vi "configuration UI.vi"() -> ()   [LabVIEW 2013, in "user tag bus module editor node.lvclass"]
uses:
  user tag bus module editor node.lvclass
  <vilib>/CEF_TreeControl/Node/NodeRef.ctl
  <vilib>/CEF_TreeControl/Node/NISE_CEF_Node.lvclass
  <vilib>/NI/AMC/Message Queue.ctl
  <vilib>/NI/AMC/Message.ctl
  <vilib>/NI/Tools/Keyed Array/KeyedArray.ctl
  <vilib>/CEF_TreeControl/Node/UserEventRef.ctl
  <vilib>/CEF_TreeControl/Controls/EventCluster.ctl
  module/configuration/state module configuration.ctl
  <vilib>/NI/Tag Bus Module Framework/channel/TBM channel.lvclass
  user tag bus module editor node.lvclass/user tag bus module editor node.ctl
  <vilib>/NI/Tag Bus Module Framework/root configuration/TBM configuration.lvclass/TBM configuration.ctl
  module/configuration/user tag bus module configuration.lvclass/user tag bus module configuration.ctl
  <vilib>/NI/Tag Bus Module Framework/root configuration/create GUID.vi
  module/configuration/user tag bus module configuration.lvclass
  <vilib>/CEF_TreeControl/NISE_CEF_TreeControl.lvlib
  Configuration Editor/Classes/Engine Parent/Engine Parent Editor Node.lvclass
  <vilib>/NI/Tag Bus Module Framework/root configuration/TBM configuration.lvclass
  <vilib>/NI/Tools/Keyed Array/Tools_KeyedArray.lvlib
  <vilib>/NI/AMC/AMC.lvlib
panel:
  in  "Tab Control":enum32{"Static State Configuration"}(tab)
  in  "Output Tag":u16(ring)
  in  "Input Tag":u16(ring)
  in  "Initial State":u8
  in  "user event":T1
  in  "main queue":T2
  in  "node ref":T3
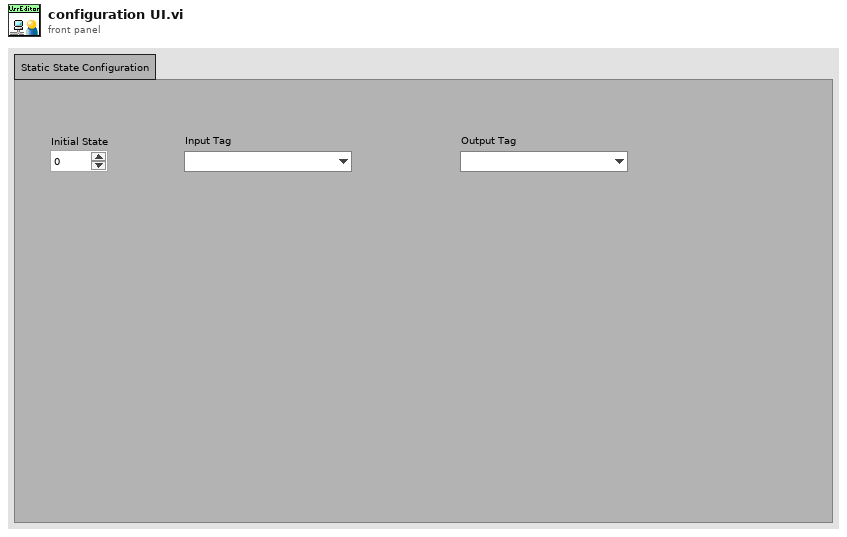
[diagram p1: front panel]
types:
  T1 = typedef "NISE_CEF_Node.lvclass/UserEventRef.ctl" = refnum<user-event>
  T2 = typedef "AMC.lvlib/Message Queue.ctl" = refnum<queue>
  T3 = typedef "NISE_CEF_Node.lvclass/NodeRef.ctl" = refnum<data-value>
  T4 = typedef "NISE_CEF_TreeControl.lvlib/EventCluster.ctl" = cluster{"command":string, "data":string}
  T5 = typedef "user tag bus module configuration.lvclass/state module configuration.ctl" = cluster{"fixed input":refnum<class "TBM channel.lvclass">, "fixed output":refnum<class "TBM channel.lvclass">, "initial state":u8}
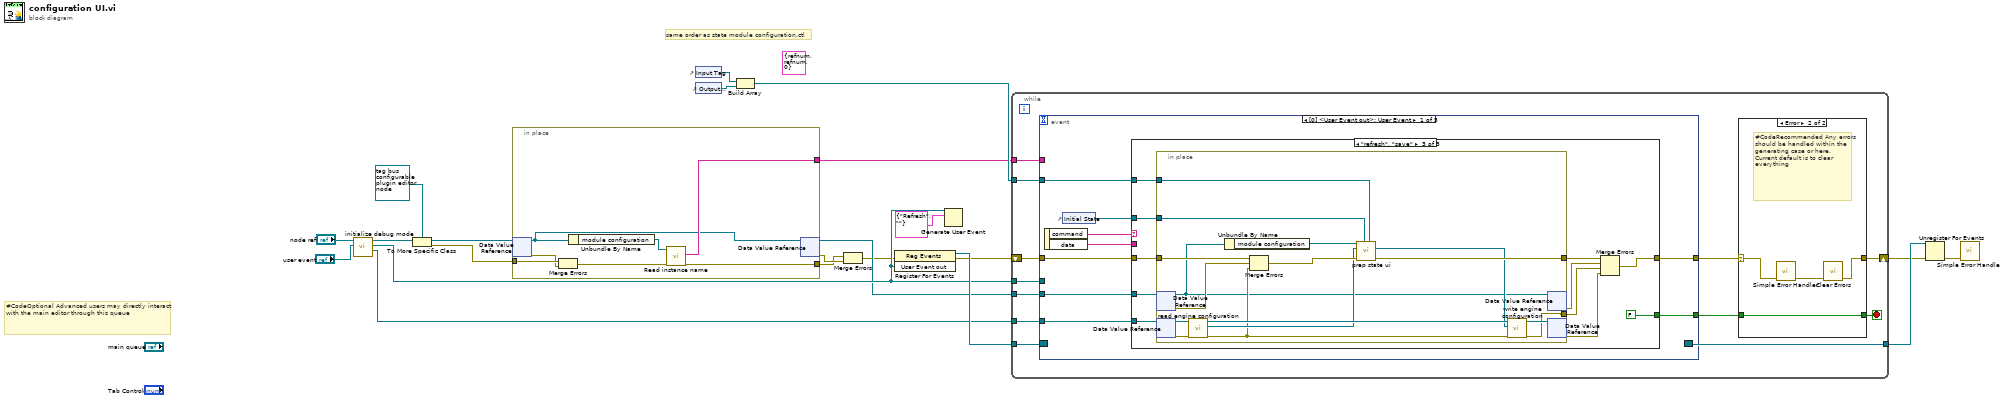
[diagram p0: block diagram]
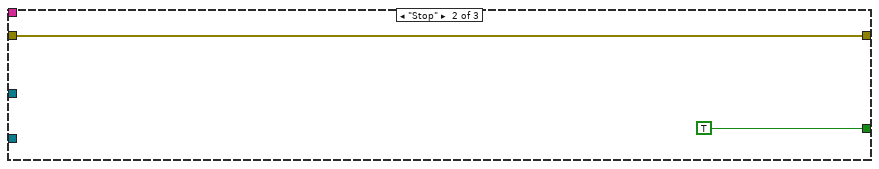
[diagram p4: hidden frame]
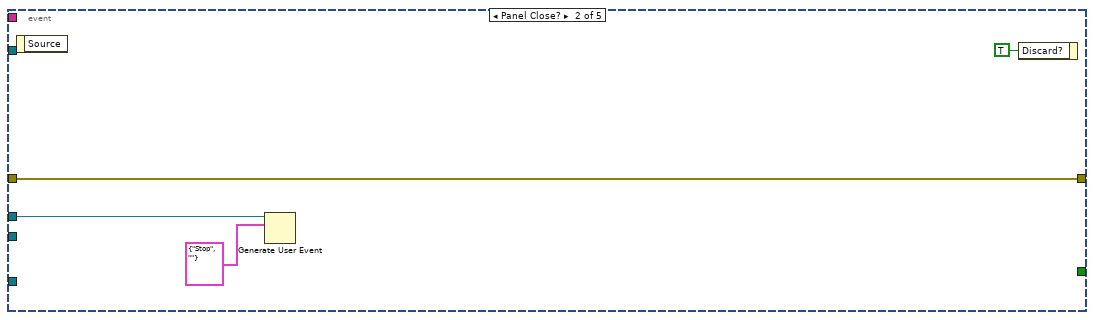
[diagram p5: hidden frame]
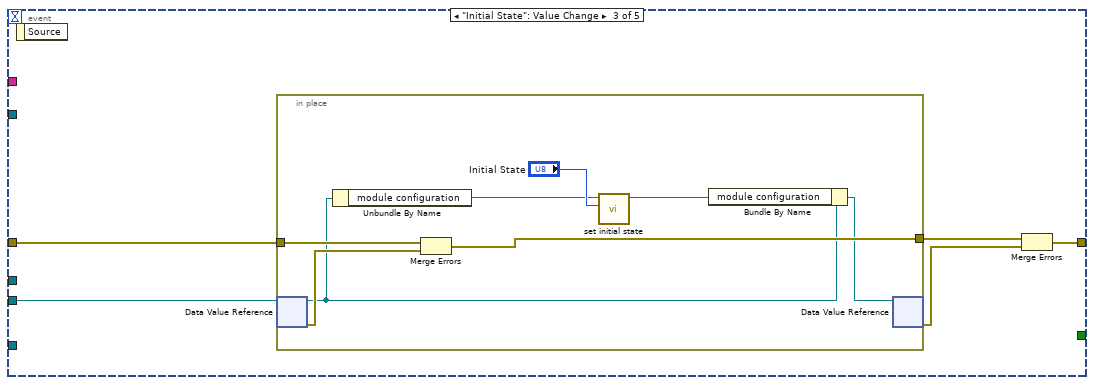
[diagram p6: hidden frame]
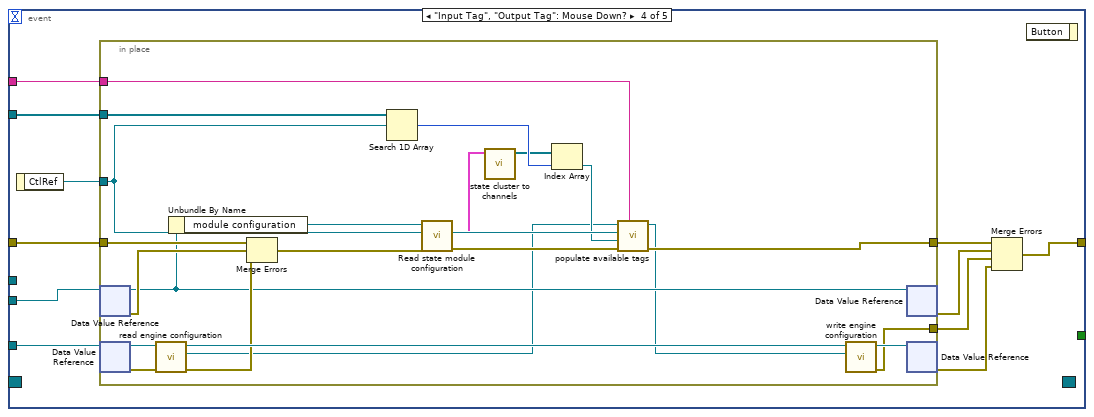
[diagram p7: hidden frame]
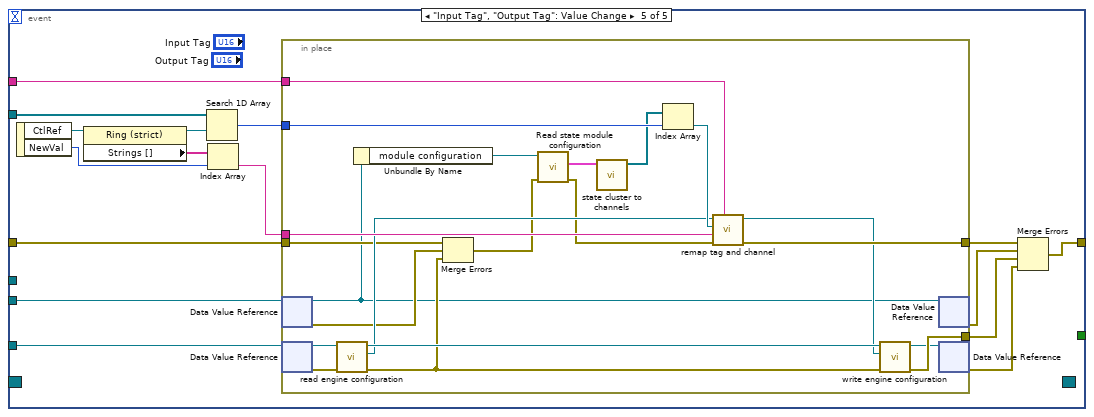
[diagram p8: hidden frame]
diagram:
  (unwired) T5 {"fixed input"=refnum, "fixed output"=refnum, "initial state"=0} ("state module configuration")
  # "same order as state module configuration.ctl"
  # "#CodeOptional Advanced users may directly interact with the main editor through this queue"
  n1 = call "initialize debug mode.vi"("User Event in"="user event", "editor node in"="node ref") -> ("engine"=w13:refnum<data-value>, "User Event out"=w9:T1, "editor node out"=w16:T3)  [unwired: 7 in]
  n2 = To More Specific Class(target class=refnum<data-value> refnum ("data value reference"), reference=w16) -> (specific class reference=w7:refnum<data-value>, error out=w3:errorcluster)  [unwired: 1 in]
  n3 = in-place {
    in-place-border: w3 -> [w29]
    in-place-border: [w26] -> w2
    in-place-border: [w25] -> w1
    n4 = in-place-dvr #1(w7) -> (w23:refnum<class "user tag bus module editor node.lvclass">, w28:errorcluster)
    n5 = Merge Errors(w29, w28) -> (w27:errorcluster)
    n6 = Unbundle By Name(w23) -> ("module configuration"=w24:refnum<class "user tag bus module configuration.lvclass">)
    n7 = call <vilib>:"Read instance name.vi"("error in"=w27, "configuration in"=w24) -> ("error out"=w26:errorcluster, "instance id"=w25:string)  [unwired: 7 in, 1 out]
    n8 = in-place-dvr #1(w23) -> (w6:refnum<data-value>, w5:errorcluster)
  }
  n9 = control-ref of="Input Tag"() -> (w11:refnum<vi>)
  n10 = control-ref of="Output Tag"() -> (w12:refnum<vi>)
  n11 = Build Array(w11, w12) -> (w10:refnum<vi>[])
  n12 = Merge Errors(w2, w5) -> (w4:errorcluster)
  n13 = register-events(error in=w4, w9) -> (reference out=w22:refnum<event-registration>, error out=w18:errorcluster)  [unwired: 1 in]
  n14 = Generate User Event(user event=w9, event data cluster=T4 {"command"="Refresh", "data"=""} ("event data")) -> ()  [unwired: 2 in, 2 out]
  n15 = while {
    tunnel: w22 -> [w41]
    tunnel: [w40] -> w21
    shift-right: [w36] -> w20
    shift-left: w18 -> [w39]
    tunnel: w1 -> [w35]
    tunnel: w6 -> [w34]
    tunnel: w13 -> [w33]
    tunnel: w10 -> [w32]
    tunnel: w9 -> [w31]
    stop <- w37 stop-if-true
    n16 = event shown="[0] <User Event out>: User Event" {
      selector: w41 -> [_ _ _ _ _]
      dyn-events: [_ _ _ _ _] -> w40
      timeout: _ -> [_ _ _ _ _]
      tunnel: [w54 _ _ _ _] -> w30
      tunnel: [w55 w90 w93 w109 w143] -> w38
      tunnel: w39 -> [w56 w90 w94 w110 w137]
      tunnel: w35 -> [_ _ _ w113 w149]
      tunnel: w34 -> [w52 _ w95 w107 w141]
      tunnel: w33 -> [w51 _ _ w108 w142]
      tunnel: w32 -> [w48 _ _ w112 w147]
      tunnel: w31 -> [_ w88 _ _ _]
      event User Event {
        n17 = event-data() -> ("command"=w53:string, "data"=w50:string)  [unwired: 1 in]
        n18 = control-ref of="Initial State"() -> (w49:refnum<vi>)
        n19 = case shown="\"refresh\", \"save\"" w53 {
          tunnel: [_ TRUE FALSE] -> w54
          tunnel: w51 -> [_ _ w65]
          tunnel: w56 -> [w57 w58 w69]
          tunnel: [w57 w58 w63] -> w55
          tunnel: w52 -> [_ _ w64]
          tunnel: w50 -> [_ _ _]
          tunnel: w49 -> [_ _ w67]
          tunnel: w48 -> [_ _ w66]
          frame Default {
          }
          frame "Stop" {
          }
          frame "refresh", "save" {
            n20 = in-place {
              in-place-border: w69 -> [w86]
              in-place-border: [w85] -> w68
              in-place-border: w67 -> [w84]
              in-place-border: w66 -> [w83]
              in-place-border: [w80] -> w60
              n21 = in-place-dvr #2(w64) -> (w72:refnum<class "user tag bus module editor node.lvclass">, w73:errorcluster)
              n22 = in-place-dvr #3(w65) -> (w79:refnum<class "Engine Parent Editor Node.lvclass">, w78:errorcluster)
              n23 = call "read engine configuration.vi"("error in"=w78, "Engine Parent Editor Node in"=w79) -> ("error out"=w74:errorcluster, "engine configuration"=w75:refnum<class "engine configuration.lvclass">, "Engine Parent Editor Node out"=w77:refnum<class "Engine Parent Editor Node.lvclass">)  [unwired: 7 in]
              n24 = Unbundle By Name(w72) -> ("module configuration"=w71:refnum<class "user tag bus module configuration.lvclass">)
              n25 = Merge Errors(w86, w73, w74) -> (w82:errorcluster)
              n26 = call "prep state ui.vi"("tag references"=w83, "Initial State"=w84, "error in"=w82, "engine configuration in"=w75, "user tag bus module configuration in"=w71) -> ("error out"=w85:errorcluster, "engine configuration out"=w76:refnum<class "engine configuration.lvclass">)  [unwired: 5 in]
              n27 = call "write engine configuration.vi"("error in"=w74, "engine configuration"=w76, "Engine Parent Editor Node in"=w77) -> ("error out"=w80:errorcluster, "Engine Parent Editor Node out"=w81:refnum<class "Engine Parent Editor Node.lvclass">)  [unwired: 7 in]
              n28 = in-place-dvr #2(w72) -> (w61:errorcluster)  [unwired: 1 out]
              n29 = in-place-dvr #3(w81) -> (w62:errorcluster)  [unwired: 1 out]
            }
            n30 = Merge Errors(w68, w61, w60, w62) -> (w63:errorcluster)
          }
        }
      }
      event Panel Close? {
        n31 = event-data() -> ()  [unwired: 1 in, 1 out]
        n32 = Generate User Event(user event=w88, event data cluster=T4 {"command"="Stop", "data"=""} ("event data")) -> ()  [unwired: 2 in, 2 out]
        n33 = event-data("Discard?"=TRUE) -> ()  [unwired: 1 in, 1 out]
      }
      event "Initial State": Value Change {
        n34 = event-data() -> ()  [unwired: 1 in, 1 out]
        n35 = in-place {
          in-place-border: w94 -> [w102]
          in-place-border: [w101] -> w92
          n36 = in-place-dvr #4(w95) -> (w99:refnum<class "user tag bus module editor node.lvclass">, w100:errorcluster)
          n37 = Unbundle By Name(w99) -> ("module configuration"=w97:refnum<class "user tag bus module configuration.lvclass">)
          n38 = Merge Errors(w102, w100) -> (w101:errorcluster)
          n39 = call "set initial state.vi"("state module configuration.initial state"="Initial State", "tag bus configurable plugin module configuration in"=w97) -> ("tag bus configurable plugin module configuration out"=w96:refnum<class "user tag bus module configuration.lvclass">)  [unwired: 9 in]
          n40 = Bundle By Name(cluster=w99, "module configuration"=w96) -> (w98:refnum<class "user tag bus module editor node.lvclass">)
          n41 = in-place-dvr #4(w98) -> (w91:errorcluster)  [unwired: 1 out]
        }
        n42 = Merge Errors(w92, w91) -> (w93:errorcluster)
      }
      event "Input Tag", "Output Tag": Mouse Down? {
        n43 = event-data() -> ("CtlRef"=w111:refnum<vi>)  [unwired: 1 in]
        n44 = in-place {
          in-place-border: [w136] -> w114
          in-place-border: w113 -> [w135]
          in-place-border: w112 -> [w134]
          in-place-border: w111 -> [w133]
          in-place-border: w110 -> [w127]
          in-place-border: [w119] -> w105
          n45 = in-place-dvr #5(w107) -> (w118:refnum<class "user tag bus module editor node.lvclass">, w120:errorcluster)
          n46 = in-place-dvr #6(w108) -> (w125:refnum<class "Engine Parent Editor Node.lvclass">, w122:errorcluster)
          n47 = call "read engine configuration.vi"("error in"=w122, "Engine Parent Editor Node in"=w125) -> ("error out"=w121:errorcluster, "engine configuration"=w115:refnum<class "engine configuration.lvclass">, "Engine Parent Editor Node out"=w124:refnum<class "Engine Parent Editor Node.lvclass">)  [unwired: 7 in]
          n48 = Unbundle By Name(w118) -> ("module configuration"=w117:refnum<class "user tag bus module configuration.lvclass">)
          n49 = Merge Errors(w127, w120, w121) -> (w126:errorcluster)
          n50 = Search 1D Array(1D array=w134, element=w133) -> (index of element=w132:i32)  [unwired: 1 in]
          n51 = call "Read state module configuration.vi"("error in"=w126, "user tag bus module configuration In"=w117) -> ("error out"=w128:errorcluster, "state module configuration"=w129:T5)  [unwired: 7 in, 1 out]
          n52 = call "state cluster to channels.vi"("state module configuration"=w129) -> ("channels"=w131:refnum<class "TBM channel.lvclass">[])  [unwired: 10 in]
          n53 = Index Array(array=w131, index=w132) -> (element=w130:refnum<class "TBM channel.lvclass">)
          n54 = call "populate available tags.vi"("instance id"=w135, "error in"=w128, "channel"=w130, "CtlRef"=w133, "engine configuration in"=w115) -> ("error out"=w136:errorcluster, "engine configuration out"=w116:refnum<class "engine configuration.lvclass">)  [unwired: 5 in]
          n55 = call "write engine configuration.vi"("engine configuration"=w116, "Engine Parent Editor Node in"=w124) -> ("error out"=w119:errorcluster, "Engine Parent Editor Node out"=w123:refnum<class "Engine Parent Editor Node.lvclass">)  [unwired: 8 in]
          n56 = in-place-dvr #5(w118) -> (w106:errorcluster)  [unwired: 1 out]
          n57 = in-place-dvr #6(w123) -> (w104:errorcluster)  [unwired: 1 out]
        }
        n58 = Merge Errors(w114, w106, w105, w104) -> (w109:errorcluster)
        n59 = event-data() -> ()  [unwired: 2 in, 1 out]
      }
      event "Input Tag", "Output Tag": Value Change {
        n60 = event-data() -> ("CtlRef"=w152:refnum<vi>, "NewVal"=w145:u16)  [unwired: 1 in]
        n61 = property on="Property Node" class="Ring (strict)"(reference=w152) -> (reference out=w146:refnum<vi>, "Strings []"=w151:string[])  [unwired: 1 in, 1 out]
        n62 = Search 1D Array(1D array=w147, element=w146) -> (index of element=w144:i32)  [unwired: 1 in]
        n63 = Index Array(array=w151, index=w145) -> (element=w148:string)
        n64 = in-place {
          in-place-border: [w173] -> w150
          in-place-border: w149 -> [w172]
          in-place-border: w148 -> [w171]
          in-place-border: w144 -> [w170]
          in-place-border: [w165] -> w140
          in-place-border: w137 -> [w160]
          n65 = in-place-dvr #7(w141) -> (w153:refnum<class "user tag bus module editor node.lvclass">, w158:errorcluster)
          n66 = in-place-dvr #8(w142) -> (w167:refnum<class "Engine Parent Editor Node.lvclass">, w166:errorcluster)
          n67 = call "read engine configuration.vi"("error in"=w166, "Engine Parent Editor Node in"=w167) -> ("error out"=w159:errorcluster, "engine configuration"=w162:refnum<class "engine configuration.lvclass">, "Engine Parent Editor Node out"=w163:refnum<class "Engine Parent Editor Node.lvclass">)  [unwired: 7 in]
          n68 = Unbundle By Name(w153) -> ("module configuration"=w156:refnum<class "user tag bus module configuration.lvclass">)
          n69 = Merge Errors(w160, w158, w159) -> (w157:errorcluster)
          n70 = call "Read state module configuration.vi"("error in"=w157, "user tag bus module configuration In"=w156) -> ("error out"=w155:errorcluster, "state module configuration"=w154:T5)  [unwired: 7 in, 1 out]
          n71 = call "state cluster to channels.vi"("state module configuration"=w154) -> ("channels"=w169:refnum<class "TBM channel.lvclass">[])  [unwired: 10 in]
          n72 = Index Array(array=w169, index=w170) -> (element=w168:refnum<class "TBM channel.lvclass">)
          n73 = call "remap tag and channel.vi"("instance id"=w172, "error in"=w155, "tag name"=w171, "channel"=w168, "engine configuration in"=w162) -> ("error out"=w173:errorcluster, "engine configuration out"=w161:refnum<class "engine configuration.lvclass">)  [unwired: 5 in]
          n74 = call "write engine configuration.vi"("error in"=w159, "engine configuration"=w161, "Engine Parent Editor Node in"=w163) -> ("error out"=w165:errorcluster, "Engine Parent Editor Node out"=w164:refnum<class "Engine Parent Editor Node.lvclass">)  [unwired: 7 in]
          n75 = in-place-dvr #7(w153) -> (w139:errorcluster)  [unwired: 1 out]
          n76 = in-place-dvr #8(w164) -> (w138:errorcluster)  [unwired: 1 out]
        }
        n77 = Merge Errors(w150, w139, w140, w138) -> (w143:errorcluster)
      }
    }
    n78 = case shown="Error" w38 {
      selector: w38 -> [w42 w46]
      tunnel: [w43 w47] -> w37
      tunnel: w30 -> [w43 w47]
      tunnel: [w42 w44] -> w36
      frame No Error {
      }
      frame Error {
        # "#CodeRecommended Any errors should be handled within the generating case or here. Current default is to clear everything"
        n79 = call <vilib>:"Simple Error Handler.vi"("error in (no error)"=w46) -> ("error out"=w45:errorcluster)  [unwired: 4 in, 4 out]
        n80 = call <vilib>:"Clear Errors.vi"("error in (no error)"=w45) -> ("error out"=w44:errorcluster)  [unwired: 6 in]
      }
    }
  }
  n81 = Unregister For Events(event registration refnum=w21, error in=w20) -> (error out=w17:errorcluster)
  n82 = call <vilib>:"Simple Error Handler.vi"("error in (no error)"=w17) -> ()  [unwired: 4 in, 5 out]
